vi "main_xyz.vi"() -> ()   [LabVIEW 2018]
uses:
  <vilib>/Platform/TimedLoop/XDataNode/timing_clust.ctl
  <vilib>/Platform/TimedLoop/XDataNode/nitl_modes.ctl
  <vilib>/Platform/TimedLoop/XDataNode/wakeup.ctl
  <vilib>/Analysis/_algsub.llb/Real Vector Norm.vi
  <vilib>/FPGAPlugInAG/myRIO-1900/niLvFpga_Open_myRIO-1900.vi
  <vilib>/rvi/interface/common/dynamic/niFpgaDynamicAddResources.vi
  <vilib>/Utility/error.llb/Error Cluster From Error Code.vi
  <vilib>/rvi/errors/niLvFpgaAdjustHostInterfaceError.vi
  <vilib>/rvi/interface/nirviOpenFPGA/nirviOpenFPGA.xnode
  FPGA Bitfiles/STW_FPGATarget_motercontrol_I8R9CeC8UVc.lvbitx
  motercontrol.vi
  <vilib>/Platform/TimedLoop/XDataNode/XDataNode.xnode
  <vilib>/rvi/interface/nirviReadWriteControl/nirviReadWriteControl.xnode
  <vilib>/Platform/TimedLoop/XDataNode/XDNodeRunTimeDep.lvlib
  NiFpgaLv.dll
  <vilib>/rvi/interface/Simulation/niFpgaSimulationCallBeginRW.vi
  <vilib>/Analysis/NI_AALPro.lvlib
panel:
  out "length":dbl[](array[numeric])
  out "Array 2":dbl[](array[numeric])
  in  "down":bool
  in  "up":bool
  out "long length_max":dbl
  in  "long length_min":dbl
  out "Array":dbl[][](array[numeric])
  in  "range":dbl=30.0
  out "out len 3":dbl
  out "out len 2":dbl
  out "out len 1":dbl
  out "length_max":dbl=112.0
  in  "length_min":dbl=82.0
  in  "Y":dbl
  in  "Z":dbl=100.0
  in  "X":dbl
  out "Duty Cycle 3":dbl(slide) scale=0.0..1.0
  out "Duty Cycle 2":dbl(slide) scale=0.0..1.0
  in  "Period (Ticks)":u32=100
  out "Duty Cycle":dbl(slide) scale=0.0..1.0
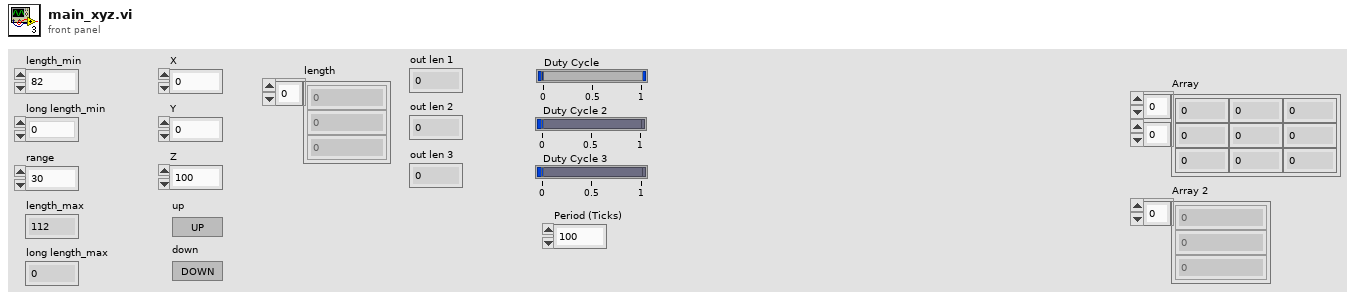
[diagram p1: front panel]
types:
  T1 = typedef "XDNodeRunTimeDep.lvlib/timing_clust.ctl" = cluster{"Expected End [f-1]":u64, "Actual End [f-1]":u64, "Finished Late? [f-1]":bool, "Expected End [i-1]":u64, "Actual End [i-1]":u64, "Finished Late? [i-1]":bool, "Expected Start [i]":u64, "Actual Start [i]":u64, "Expected Start [f]":u64, "Actual Start [f]":u64, "Source Name":string, "Structure Name":string, "Period":i64, "Deadline":i64, "Offset":i64, "Start":i64, "Priority":i32, "Timeout":i32, "Mode":T2, "Wakeup Reason":T3, "Error":errorcluster, "Source Type":string, "Secondary Source Type":string, "Global End Time":u64, "Global Start Time":u64, "Frame Duration":u64, "Iteration Duration":u64, "Assigned CPU":i32, "I/O Scan Engine Mode":u32}
  T2 = typedef "XDNodeRunTimeDep.lvlib/nitl_modes.ctl" = enum32{"No Change", "Process missed periods, maintain original phase", "Discard missed periods, maintain original phase", "Process missed periods, ignore original phase", "Discard missed periods, ignore original phase"}
  T3 = typedef "XDNodeRunTimeDep.lvlib/wakeup.ctl" = enum32{"Normal", "Aborted", "Asynchronous wakeup", "Timing source error", "Timed loop error", "Timeout"}
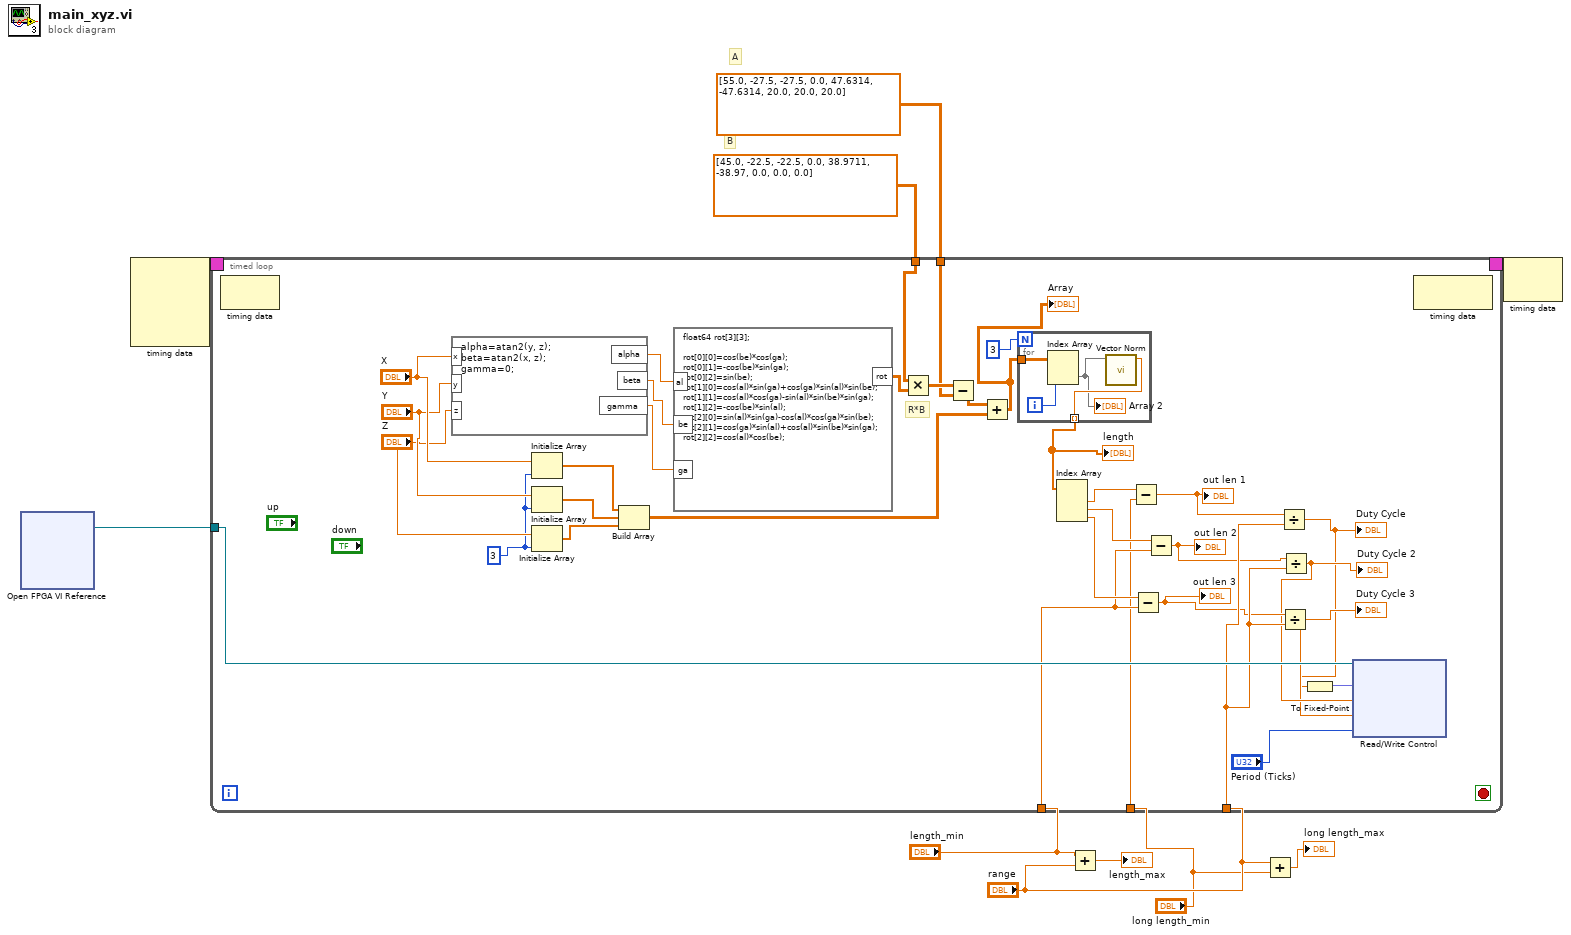
[diagram p0: block diagram]
diagram:
  # "A"
  # "B"
  n1 = xnode "Open FPGA VI Reference"() -> ("FPGA VI Reference Out"=w8:refnum<k20>)  [unwired: 2 in, 1 out]
  n2 = node-c288() -> (w10:T1)  [unwired: 4 in]
  n3 = timed-loop {
    timing: w10 -> [_]
    timing-out: [_] -> w9
    tunnel: w8 -> [w44]
    tunnel: dbl[][] [[55.0, -27.5, -27.5], [0.0, 47.6314, -47.6314], [20.0, 20.0, 20.0]] -> [w40]
    tunnel: dbl[][] [[45.0, -22.5, -22.5], [0.0, 38.9711, -38.97], [0.0, 0.0, 0.0]] -> [w42]
    tunnel: "length_min" -> [w33]
    tunnel: "range" -> [w31]
    tunnel: "long length_min" -> [w14]
    stop <- _ stop-if-true
    w23 = 3
    # "R*B"
    n4 = node-c288() -> ()  [unwired: 1 in, 1 out]
    n5 = formula code="alpha=atan2(y, z);\nbeta=atan2(x, z);\ngamma=0;"("x"="X", "y"="Y", "z"="Z") -> ("alpha"=w39:dbl, "beta"=w38:dbl, "gamma"=w37:dbl)
    n6 = Initialize Array("X", w23) -> (w20:dbl[])
    n7 = Initialize Array("Y", w23) -> (w21:dbl[])
    n8 = Initialize Array("Z", w23) -> (w22:dbl[])
    n9 = Build Array(w20, w21, w22) -> (w19:dbl[][])
    n10 = formula code="float64 rot[3][3];\n\nrot[0][0]=cos(be)*cos(ga);\nrot[0][1]=-cos(be)*sin(ga);\nrot[0][2]=sin(be);\nrot[1][0]=cos(al)*sin(ga)+cos(ga)*sin(al)*sin(be);\nrot[1][1]=cos(al)*cos(ga)-sin(al)*sin(be)*sin(ga);\nrot[1][2]=-cos(be)*sin(al);\nrot[2][0]=sin(al)*sin(ga)-cos(al)*cos(ga)*sin(be);\nrot[2][1]=cos(ga)*sin(al)+cos(al)*sin(be)*sin(ga);\nrot[2][2]=cos(al)*cos(be);"("al"=w39, "be"=w38, "ga"=w37) -> ("rot"=w13:dbl[][])
    n11 = Multiply(x=w42, y=w13) -> (x*y=w41:dbl[][])
    n12 = Subtract(x=w41, y=w40) -> (x-y=w27:dbl[][])
    n13 = Add(x=w27, y=w19) -> (x+y=w12:dbl[][])
    "Array" <- w12
    n14 = for {
      N: 3 -> [_]
      tunnel: w12 -> [w48]
      tunnel: [w46] -> w11 mode=indexing
      i -> [w47]
      n15 = Index Array(array=w48, index (col)=w47) -> (element=w45:dbl[])  [unwired: 1 in]
      "Array 2" <- w45
      n16 = call-poly <vilib>:"Vector Norm.vi"("Input Vector"=w45) -> ("norm"=w46:dbl)  [unwired: 9 in, 1 out]
    }
    "length" <- w11
    n17 = Index Array(array=w11) -> (element #1=w36:dbl, element #2=w35:dbl, element #3=w34:dbl)  [unwired: 3 in]
    n18 = Subtract(x=w36, y=w14) -> (x-y=w30:dbl)
    "out len 1" <- w30
    n19 = Subtract(x=w34, y=w33) -> (x-y=w28:dbl)
    "out len 3" <- w28
    n20 = Subtract(x=w35, y=w33) -> (x-y=w29:dbl)
    "out len 2" <- w29
    n21 = Divide(x=w30, y=w31) -> (x/y=w15:dbl)
    "Duty Cycle" <- w15
    n22 = Divide(x=w28, y=w31) -> (x/y=w17:dbl)
    "Duty Cycle 3" <- w17
    n23 = Divide(x=w29, y=w31) -> (x/y=w18:dbl)
    "Duty Cycle 2" <- w18
    n24 = To Fixed-Point(number=w15) -> (fixed-point=w16:fxp<+/-,32,16>)  [unwired: 1 in]
    n25 = xnode "Read/Write Control"("FPGA VI Reference In"=w44, "Duty Cycle"=w16, "Duty Cycle 2"=w18, "Duty Cycle 3"=w17, "Period (Ticks)"="Period (Ticks)") -> ()  [unwired: 1 in, 2 out]
    n26 = node-c288() -> ()  [unwired: 1 in, 1 out]
  }
  n27 = Add(x="length_min", y="range") -> (x+y=→"length_max":dbl)
  n28 = Add(x="range", y="long length_min") -> (x+y=→"long length_max":dbl)
  n29 = node-c288(w9) -> ()  [unwired: 1 out]
